vi "ASIC_SET_SUM_NEW.vi"(0 "connection ID":refnum<k5>, 1 "Channel Enable":i32(slide) scale=0.0..6.0, 2 "Attenuation Select":i32(slide) scale=0.0..15.0, 3 "Clipping Select":i32(slide)=3 scale=1.0..3.0, 4 "Ib Clip select":i32(slide)=63 scale=0.0..63.0, 5 "error in":errorcluster) -> (14 "connection ID out":refnum<k5>, 19 "error out":errorcluster)   [LabVIEW 2012]
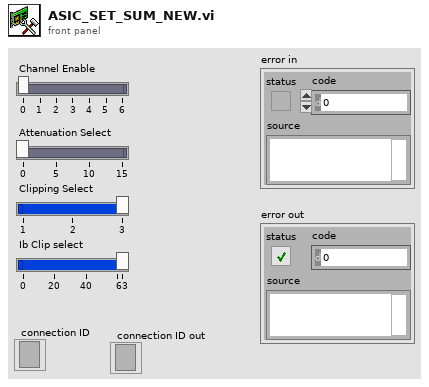
[diagram p1: front panel]
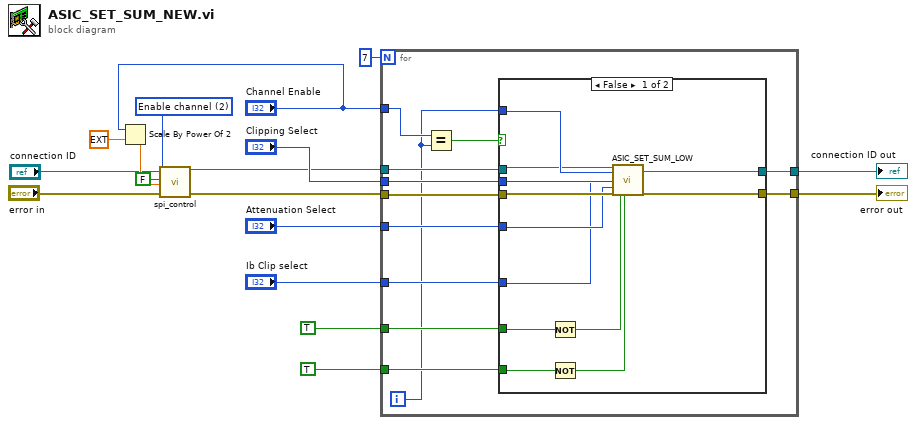
[diagram p0: block diagram]
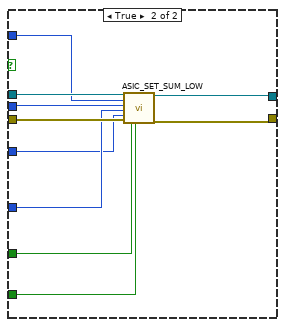
[diagram p2: hidden frame]
diagram:
  w11 = u16 2 items=["Attenuation", "Clipping", "Enable channel", "Delay line", "ASIC"] ("Device")
  n1 = Scale By Power Of 2(n="Channel Enable", x=ext 1.0) -> (x*2^n=w9:ext)
  n2 = call "spi_control.vi"("connection ID"="connection ID", "Device"=w11, "Read/#write"=FALSE, "Data"=w9, "error out 3"="error in") -> ("connection ID out"=w6:refnum<k5>, "error out 2"=w7:errorcluster)  [unwired: 7 in, 6 out]
  n3 = for {
    N: 7 -> [_]
    tunnel: "Clipping Select" -> [w29]
    tunnel: "Ib Clip select" -> [w28]
    tunnel: "Attenuation Select" -> [w27]
    tunnel: w7 -> [w26]
    tunnel: w6 -> [w25]
    tunnel: [w24] -> w2
    tunnel: [w23] -> w1
    tunnel: "Channel Enable" -> [w19]
    tunnel: TRUE ("Clip_en_b") -> [w22]
    tunnel: TRUE ("Att_en_b") -> [w21]
    i -> [w18]
    n4 = Equal?(x=w19, y=w18) -> (x = y?=w20:bool)
    n5 = case shown="False" w20 {
      tunnel: w29 -> [w37 w44]
      tunnel: w28 -> [w34 w45]
      tunnel: w27 -> [w35 w42]
      tunnel: w26 -> [w36 w51]
      tunnel: w25 -> [w38 w49]
      tunnel: [w40 w50] -> w24
      tunnel: [w41 w48] -> w23
      tunnel: w18 -> [w39 w43]
      tunnel: w22 -> [w33 w47]
      tunnel: w21 -> [w32 w46]
      frame False {
        n6 = Not(x=w33) -> (.not. x?=w31:bool)
        n7 = Not(x=w32) -> (.not. x?=w30:bool)
        n8 = call "ASIC_SET_SUM_LOW.vi"("connection ID"=w38, "Channel"=w39, "Clip_sel_b"=w37, "Ib_ClipVb"=w34, "Att gain"=w35, "error in"=w36, "Clip_en_b"=w31, "Att_en_b"=w30) -> ("connection ID out"=w41:refnum<k5>, "error out"=w40:errorcluster)  [unwired: 8 in, 2 out]
      }
      frame True {
        n9 = call "ASIC_SET_SUM_LOW.vi"("connection ID"=w49, "Channel"=w43, "Clip_sel_b"=w44, "Ib_ClipVb"=w45, "Att gain"=w42, "error in"=w51, "Clip_en_b"=w47, "Att_en_b"=w46) -> ("connection ID out"=w48:refnum<k5>, "error out"=w50:errorcluster)  [unwired: 8 in, 2 out]
      }
    }
  }
  "error out" <- w2
  "connection ID out" <- w1
